vi "Utility Query Channel Output State.vi"(8 "error in (no error)":errorcluster {"code" format="%.0x"}, 10 "Channel Name (1)":string="1", 11 "VISA resource name":refnum<visa-resource-name>) -> (0 "error out":errorcluster {"code" format="%.0x"}, 2 "In State":bool, 3 "VISA resource name out":refnum<visa-resource-name>)   [LabVIEW 2015]
doc: "This VI returns whether the power supply is in a particular output state.\n\nA constant voltage condition occurs when the output voltage is equal to the value of the agn6700>>Basic Operation>>Voltage Level property and the current is less than or equal to the value of the agn6700>>Basic Operation>>Current Limit property.\n\nA constant current condition occurs when the output current is equal to the value of the agn6700>>Basic Operation>>Current Limit property and the agn6700>>Basic Operation>>Current Limit Behavior property is set to AGN6700_VAL_CURRENT_REGULATE.\n\nAn unregulated condition occurs when the output voltage is less than the value of the agn6700>>Basic Operation>>Voltage Level property and the current is less than the value of the agn6700>>Basic Operation>>Current Limit property.\n\nAn over-voltage condition occurs when the output voltage is equal to or greater than the value of the agn6700>>Basic Operation>>OVP Limit property and the agn6700>>Basic Operation>>OVP Enabled property is set to TRUE.\n\nAn over-current condition occurs when the output current is equal to or greater than the value of the agn6700>>Basic Operation>>Current Limit property and the agn6700>>Basic Operation>>Current Limit Behavior property is set to AGN6700_VAL_CURRENT_TRIP. \n\nWhen either an over-voltage condition or an over-current condition occurs, the power supply's output protection disables the output. If the power supply is in an over-voltage or over-current state, it does not produce power until the output protection is reset. The agn6700 Reset Output Protection.vi resets the output protection. Once the output protection is reset, the power supply resumes generating a power signal."
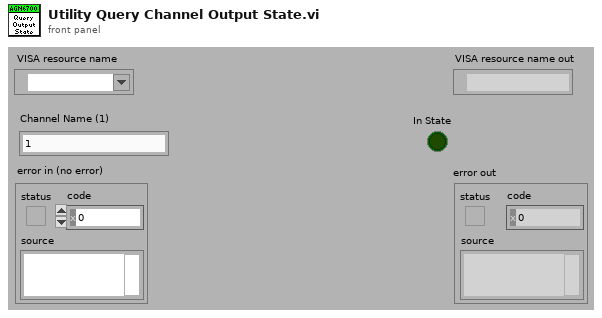
[diagram p1: front panel]
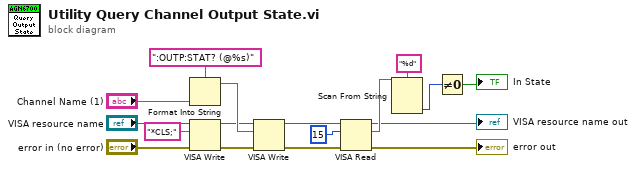
[diagram p0: block diagram]
diagram:
  n1 = Format Into String(format string=":OUTP:STAT? (@%s)", "Channel Name (1)") -> (resulting string=w11:string)  [unwired: 2 in, 1 out]
  n2 = VISA Write(VISA resource name="VISA resource name", write buffer="*CLS;", error in (no error)="error in (no error)") -> (VISA resource name out=w2:refnum<visa-resource-name>, error out=w4:errorcluster)  [unwired: 1 out]
  n3 = VISA Write(VISA resource name=w2, write buffer=w11, error in (no error)=w4) -> (VISA resource name out=w16:refnum<visa-resource-name>, error out=w15:errorcluster)  [unwired: 1 out]
  n4 = VISA Read(VISA resource name=w16, byte count=u32 15, error in (no error)=w15) -> (VISA resource name out=→"VISA resource name out":refnum<visa-resource-name>, read buffer=w14:string, error out=→"error out":errorcluster)  [unwired: 1 out]
  n5 = Scan From String(format string="%d", input string=w14) -> (output 1=w6:i32)  [unwired: 3 in, 3 out]
  n6 = Not Equal To 0?(x=w6) -> (x != 0?=→"In State":bool)
